vi "Display.vi"(6 "include timestamp? (F)":bool, 7 "prefix (\"\")":string, 8 "error in (no error)":errorcluster, 9 "clear before next write (F)":bool, 11 "log text":string) -> (0 "error out":errorcluster)   [LabVIEW 2020, in "Debug Log.lvlib"]
doc: "Use this VI to log strings generated at various points in your program. Each time you call it, it appends <b>prefix</b> + <b>log text</b> to the displayed string, optionally including a timestamp. This VI opens on first call and remains open even after the program terminates.\n\nThis VI executes even if <b>error in</b> indicates an error."
uses:
  <vilib>/Utility/Debug Log/Debug Log.lvlib
panel:
  in  "Clear before next write":bool
  out "Log":string
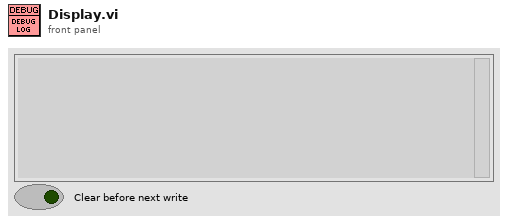
[diagram p1: front panel]
types:
  T1 = enum32{"Invalid", "Standard", "Closed", "Hidden", "Minimized", "Maximized"}
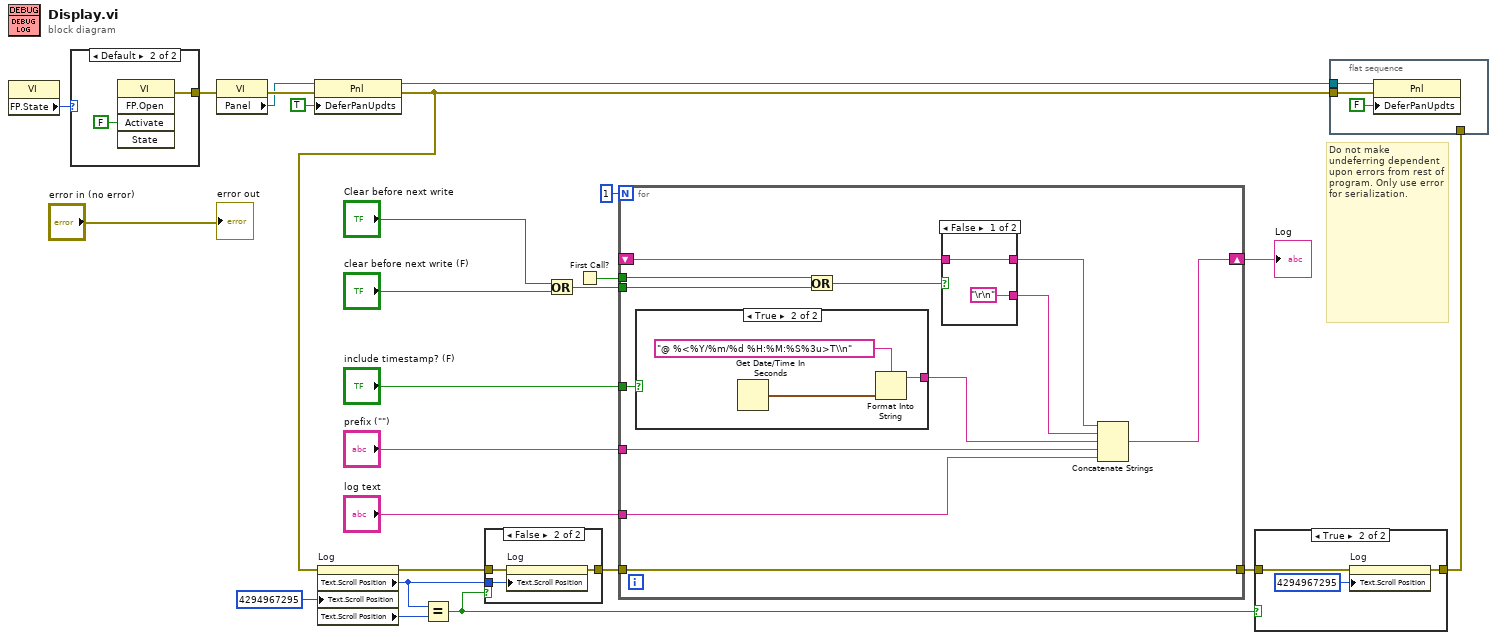
[diagram p0: block diagram]
diagram:
  # "Do not make undeferring dependent upon errors from rest of program. Only use error for serialization."
  n1 = property class="VI"() -> ("FP.State"=w18:T1)  [unwired: 2 in, 2 out]
  n2 = case shown="Default" w18 {
    tunnel: [_ w26] -> w4
    frame "Standard", "Minimized", "Maximized" {
    }
    frame Default {
      n3 = invoke class="VI" method="FP.Open"("Activate"=FALSE ("Activate?")) -> (error out=w26:errorcluster)  [unwired: 4 in, 4 out]
    }
  }
  n4 = property class="VI"(error in=w4) -> (error out=w3:errorcluster, "Panel"=w2:refnum<vi>)  [unwired: 1 in, 1 out]
  n5 = property class="Pnl"(reference=w2, error in=w3, "DeferPanUpdts"=TRUE ("Defer Panel Updates")) -> (reference out=w1:refnum<vi>, error out=w6:errorcluster)
  n6 = property on="Log" class="Str"(error in=w6, "Text.Scroll Position"=u32 4294967295) -> (error out=w13:errorcluster, "Text.Scroll Position"=w12:u32, "Text.Scroll Position"=w11:u32)  [unwired: 1 in, 1 out]
  n7 = Equal?(x=w12, y=w11) -> (x = y?=w8:bool)
  n8 = case shown="False" w8 {
    tunnel: w13 -> [w28 w31]
    tunnel: w12 -> [_ w30]
    tunnel: [w28 w29] -> w10
    frame True {
    }
    frame False {
      n9 = property on="Log" class="Str"(error in=w31, "Text.Scroll Position"=w30) -> (error out=w29:errorcluster)  [unwired: 1 in, 1 out]
    }
  }
  n10 = Or(x="Clear before next write", y="clear before next write (F)") -> (x .or. y?=w15:bool)
  n11 = First Call?() -> (First Call?: T/F=w19:bool)
  n12 = for {
    N: 1 -> [_]
    shift-right: [w43] -> w21
    shift-left: _ -> [w41]
    tunnel: "log text" -> [w39]
    tunnel: w15 -> [w38]
    tunnel: "prefix (\"\")" -> [w36]
    tunnel: "include timestamp? (F)" -> [w35]
    tunnel: w19 -> [w33]
    tunnel: w10 -> [w32]
    tunnel: [w32] -> w9
    n13 = case shown="True" w35 {
      tunnel: [_ w46] -> w34
      frame False {
      }
      frame True {
        n14 = Get Date/Time In Seconds() -> (seconds since 1Jan1904=w45:timestamp)
        n15 = Format Into String(format string="@ %<%Y/%m/%d %H:%M:%S%3u>T\\n", w45) -> (resulting string=w46:string)  [unwired: 2 in, 1 out]
      }
    }
    n16 = Or(x=w33, y=w38) -> (x .or. y?=w40:bool)
    n17 = case shown="False" w40 {
      tunnel: [w48 _] -> w42
      tunnel: w41 -> [w48 _]
      tunnel: ["\r\n" _] -> w37
      frame False {
      }
      frame True {
      }
    }
    n18 = Concatenate Strings(w42, w37, w34, w36, w39) -> (w43:string)
  }
  "Log" <- w21
  n19 = case shown="True" w8 {
    tunnel: w9 -> [w49 w51]
    tunnel: [w49 w50] -> w5
    frame False {
    }
    frame True {
      n20 = property on="Log" class="Str"(error in=w51, "Text.Scroll Position"=u32 4294967295) -> (error out=w50:errorcluster)  [unwired: 1 in, 1 out]
    }
  }
  n21 = flat-sequence {
    tunnel: w6 -> [w54]
    tunnel: w5 -> [_]
    tunnel: w1 -> [w53]
    frame #0 {
      n22 = property class="Pnl"(reference=w53, error in=w54, "DeferPanUpdts"=FALSE ("Defer Panel Updates")) -> ()  [unwired: 2 out]
    }
  }
  "error out" <- "error in (no error)"
